vi "ParseJSONBody.vi"(8 "error in (no error)":errorcluster, 11 "JSON object in":string) -> (0 "error out":errorcluster, 2 "JSON Error Strings":string[](array[string]), 3 "JSON Response Strings":string[](array[string]))   [LabVIEW 2013]
doc: "Parses the passed JSON object entry by entry. Expects the top level object to have members whose names correspond to known commands. It will extract that command to use as the condition for a case statement to pass off the processing, and extract the value of that member to pass to that command.\n\nUnknown commands return an error -375302 \"Feature not supported\""
uses:
  <vilib>/Utility/error.llb/Error Cluster From Error Code.vi
  <vilib>/regexp/Match Regular Expression.xnode
  <vilib>/ErrorRing/Error Ring.xnode
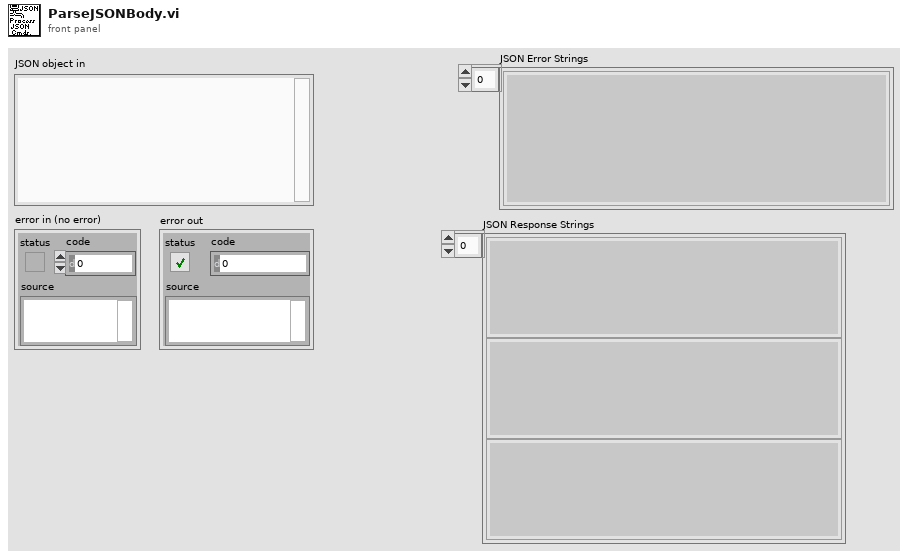
[diagram p1: front panel]
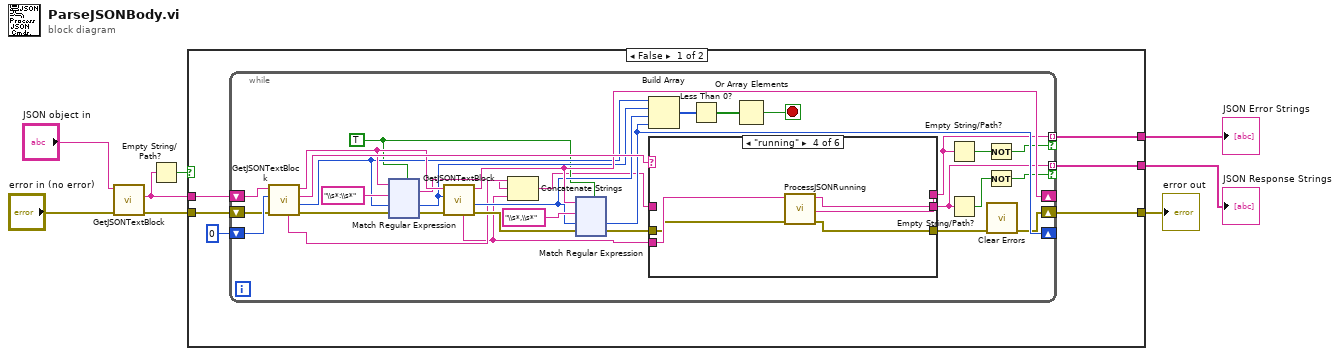
[diagram p0: block diagram]
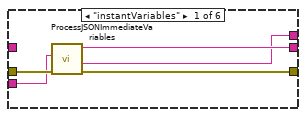
[diagram p2: hidden frame]
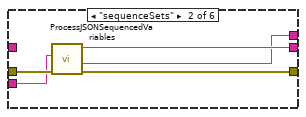
[diagram p3: hidden frame]
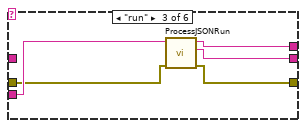
[diagram p4: hidden frame]
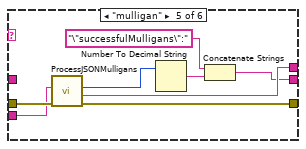
[diagram p5: hidden frame]
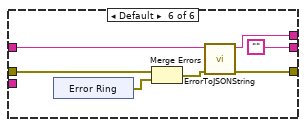
[diagram p6: hidden frame]
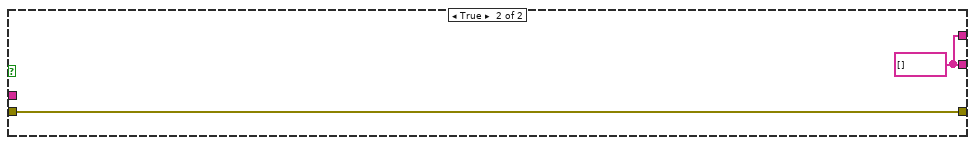
[diagram p7: hidden frame]
diagram:
  n1 = call "GetJSONTextBlock.vi"("error in (no error)"="error in (no error)", "String In"="JSON object in") -> ("error out"=w6:errorcluster, "Matched Block Contents"=w2:string)  [unwired: 5 in, 3 out]
  n2 = Empty String/Path?(string/path=w2) -> (empty?=w1:bool)
  n3 = case shown="False" w1 {
    tunnel: w6 -> [w13 w315]
    tunnel: [w12 w315] -> w5
    tunnel: [w11 w314] -> w4
    tunnel: [w10 w314] -> w3
    tunnel: w2 -> [w9 _]
    frame False {
      n4 = while {
        shift-right: [w36] -> _
        shift-left: w9 -> [w45]
        shift-right: [w32] -> _
        shift-left: 0 -> [w46]
        shift-right: [w15] -> w12
        shift-left: w13 -> [w44]
        tunnel: [w24] -> w11 mode=indexing if=w26
        tunnel: [w18] -> w10 mode=indexing if=w17
        stop <- w30 stop-if-true
        w28 = TRUE ("multiline? (F)")
        n5 = call "GetJSONTextBlock.vi"("error in (no error)"=w44, "Block Start Offset"=w46, "String In"=w45) -> ("error out"=w40:errorcluster, "Offset Past Block"=w35:i32, "Matched Block Contents"=w43:string, "String Out"=w37:string, "Matched Block"=w23:string)  [unwired: 4 in]
        n6 = xnode "Match Regular Expression"("input string"=w37, "regular expression"="\\s*:\\s*", "offset (0)"=w35, "error in"=w40, "multiline? (F)"=w28) -> ("whole match"=w22:string, "offset past match"=w34:i32, "error out"=w39:errorcluster)  [unwired: 1 in, 2 out]
        n7 = call "GetJSONTextBlock.vi"("error in (no error)"=w39, "Block Start Offset"=w34, "String In"=w37) -> ("error out"=w38:errorcluster, "Offset Past Block"=w33:i32, "String Out"=w36:string, "Matched Block"=w21:string)  [unwired: 4 in, 1 out]
        n8 = Concatenate Strings(w23, w22, w21) -> (w20:string)
        n9 = xnode "Match Regular Expression"("input string"=w36, "regular expression"="\\s*,\\s*", "offset (0)"=w33, "error in"=w38, "multiline? (F)"=w28) -> ("offset past match"=w32:i32, "error out"=w27:errorcluster)  [unwired: 1 in, 3 out]
        n10 = Build Array(w35, w34, w33, w32) -> (w31:i32[])
        n11 = case shown="\"running\"" w43 {
          tunnel: w21 -> [w278 w283 w289 w294 w300 _]
          tunnel: w27 -> [w279 w284 w288 w293 w302 w308]
          tunnel: [w277 w282 w287 w290 w301 w306] -> w16
          tunnel: [w275 w280 w286 w291 w299 w307] -> w24
          tunnel: w20 -> [_ _ _ _ _ w304]
          tunnel: [w276 w281 w285 w292 w296 ""] -> w18
          frame "instantVariables" {
            n12 = call "ProcessJSONImmediateVariables.vi"("error in (no error)"=w279, "JSON Array"=w278) -> ("error out"=w277:errorcluster, "JSON Error string"=w275:string, "JSON Response String"=w276:string)  [unwired: 6 in, 1 out]
          }
          frame "sequenceSets" {
            n13 = call "ProcessJSONSequencedVariables.vi"("error in (no error)"=w284, "JSON Array"=w283) -> ("error out"=w282:errorcluster, "JSON Error string"=w280:string, "JSON Response String"=w281:string)  [unwired: 7 in]
          }
          frame "run" {
            n14 = call "ProcessJSONRun.vi"("error in (no error)"=w288, "JSON Array"=w289) -> ("error out"=w287:errorcluster, "JSON Response String"=w285:string, "JSON Error string"=w286:string)  [unwired: 7 in]
          }
          frame "running" {
            n15 = call "ProcessJSONRunning.vi"("error in (no error)"=w293, "JSON Array"=w294) -> ("error out"=w290:errorcluster, "JSON Error string"=w291:string, "JSON Response String"=w292:string)  [unwired: 7 in]
          }
          frame "mulligan" {
            n16 = call "ProcessJSONMulligans.vi"("error in (no error)"=w302, "JSON Array"=w300) -> ("error out"=w301:errorcluster, "JSON Error string"=w299:string, "Mulligans Requested"=w298:i32)  [unwired: 7 in]
            n17 = Number To Decimal String(number=w298) -> (decimal integer string=w297:string)  [unwired: 1 in]
            n18 = Concatenate Strings("\"successfulMulligans\":" ("string"), w297) -> (w296:string)
          }
          frame Default {
            n19 = xnode "Error Ring"() -> ("error out"=w309:errorcluster)
            n20 = Merge Errors(w308, w309) -> (w305:errorcluster)
            n21 = call "ErrorToJSONString.vi"("error in (no error)"=w305, "problemJSON"=w304) -> ("error out"=w306:errorcluster, "JSON Error string"=w307:string)  [unwired: 8 in]
          }
        }
        n22 = Less Than 0?(x=w31) -> (x < 0?=w29:bool[])
        n23 = Or Array Elements(Boolean array=w29) -> (logical OR=w30:bool)
        n24 = Empty String/Path?(string/path=w24) -> (empty?=w25:bool)
        n25 = Empty String/Path?(string/path=w18) -> (empty?=w19:bool)
        n26 = Not(x=w25) -> (.not. x?=w26:bool)
        n27 = Not(x=w19) -> (.not. x?=w17:bool)
        n28 = call <vilib>:"Clear Errors.vi"("error in (no error)"=w16) -> ("error out"=w15:errorcluster)  [unwired: 6 in]
      }
    }
    frame True {
      w314 = string[] []
    }
  }
  "error out" <- w5
  "JSON Error Strings" <- w4
  "JSON Response Strings" <- w3
